vi "for_last_value.vi"() -> ()   [LabVIEW 2020]
panel:
  out "Array 2":dbl[](array[numeric])
  out "Array":i32[](array[numeric])
  out "numero \nde iteracion":i32
  # "for"
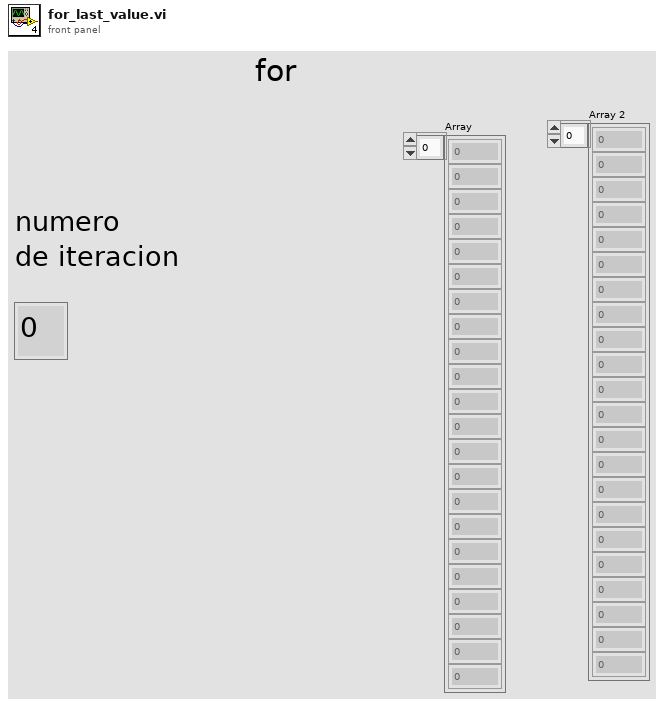
[diagram p1: front panel]
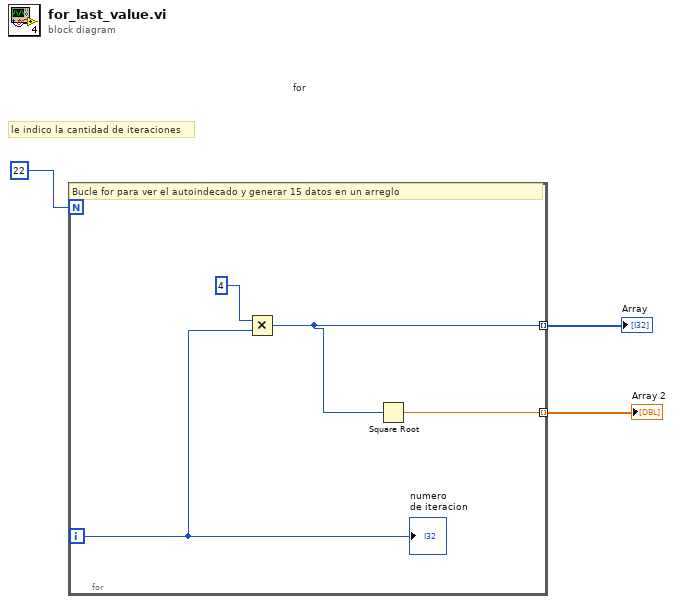
[diagram p0: block diagram]
diagram:
  # "le indico la cantidad de iteraciones"
  # "for"
  n1 = for {
    N: 22 -> [_]
    tunnel: [w5] -> w2 mode=indexing
    tunnel: [w4] -> w1 mode=indexing
    i -> [w7]
    # "Bucle for para ver el autoindecado y generar 15 datos en un arreglo"
    n2 = Multiply(x=4, y=w7) -> (x*y=w5:i32)
    n3 = Square Root(x=w5) -> (sqrt(x)=w4:dbl)
    "numero \nde iteracion" <- w7
  }
  "Array" <- w2
  "Array 2" <- w1
